vi "ID Generator.vi"() -> (1 "ID":i32)   [LabVIEW 2015]
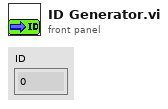
[diagram p1: front panel]
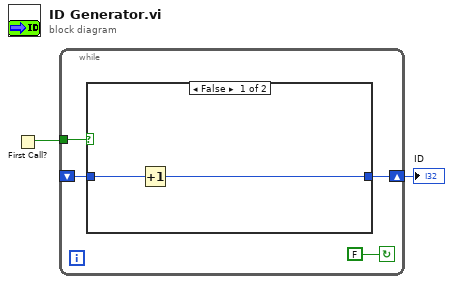
[diagram p0: block diagram]
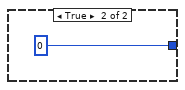
[diagram p2: hidden frame]
diagram:
  n1 = First Call?() -> (First Call?: T/F=w2:bool)
  n2 = while {
    tunnel: w2 -> [w5]
    shift-right: [w4] -> w1
    shift-left: _ -> [w3]
    stop <- FALSE continue-if-true
    n3 = case shown="False" w5 {
      tunnel: [w7 0] -> w4
      tunnel: w3 -> [w8 _]
      frame False {
        n4 = Increment(x=w8) -> (x+1=w7:i32)
      }
      frame True {
      }
    }
  }
  "ID" <- w1
